vi "drawStrokeLines.vi"(0 "picture":picture, 1 "line endpoints":cluster{"x":i16, "y":i16}[](array[cluster]), 2 "fill?(F)":bool, 3 "color(black)":u32(colorbox), 4 "stroke":T1, 5 "error in (no error)":errorcluster, 9 "strokeLength":i32=5, 11 "black in B/W?(T)":bool=TRUE) -> (14 "new picture":picture, 19 "error out":errorcluster)   [LabVIEW 2016, in "Graphics.lvclass"]
doc: "Draws multiple connected lines into a picture."
uses:
  <resource>/Framework/Providers/Open_GDS/UML/Graphics_class/Graphics.lvclass
  <resource>/Framework/Providers/Open_GDS/UML/Graphics_class/StrokeType.ctl
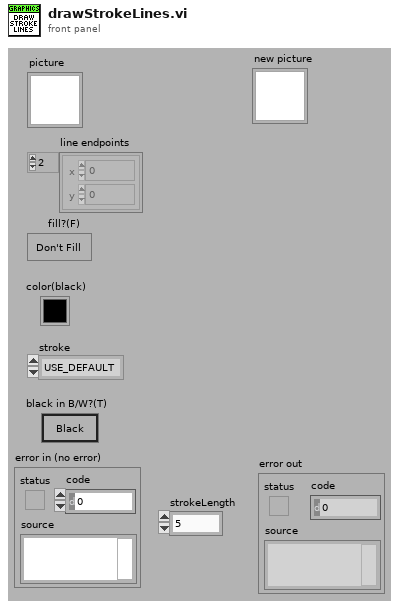
[diagram p1: front panel]
types:
  T1 = typedef "Graphics.lvclass/StrokeType.ctl" = enum16{"USE_DEFAULT", "SOLID", "DOTTED"}
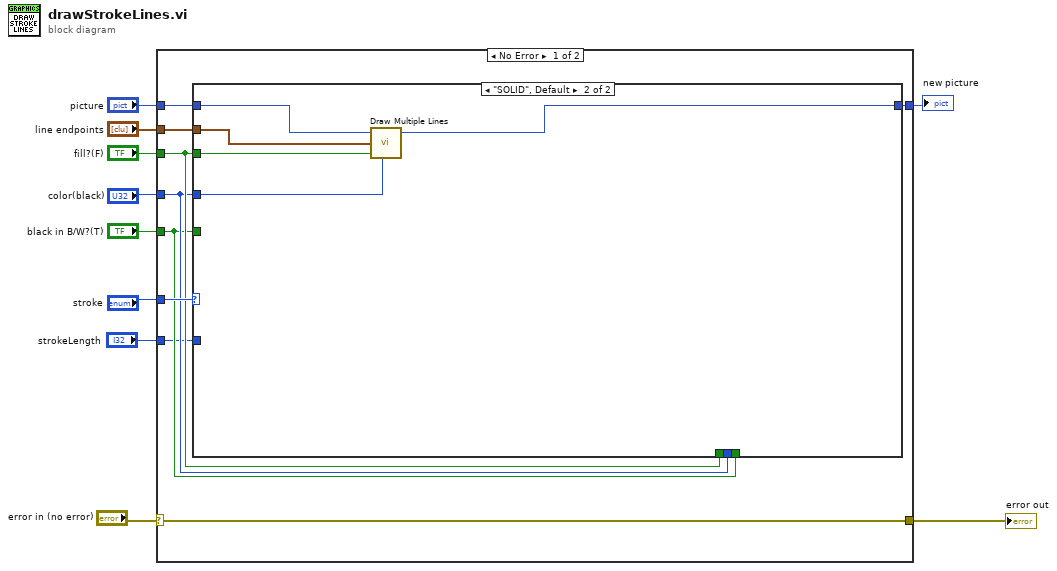
[diagram p0: block diagram]
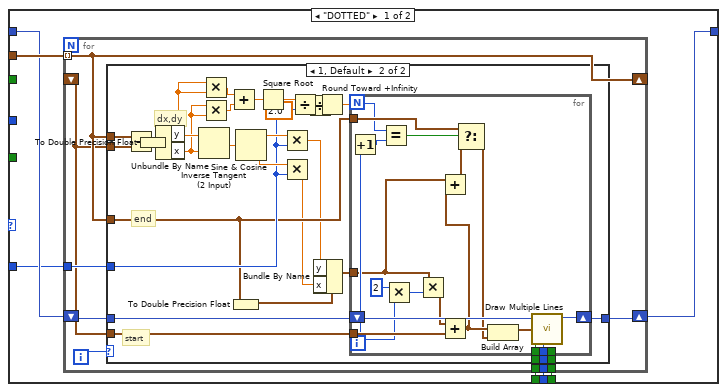
[diagram p2: hidden frame]
diagram:
  n1 = case shown="No Error" "error in (no error)" {
    selector: "error in (no error)" -> [w15 w90]
    tunnel: "picture" -> [w19 w89]
    tunnel: [w18 w89] -> w9
    tunnel: "fill?(F)" -> [w14 _]
    tunnel: "line endpoints" -> [w17 _]
    tunnel: "black in B/W?(T)" -> [w12 _]
    tunnel: "color(black)" -> [w13 _]
    tunnel: "stroke" -> [w16 _]
    tunnel: [w15 w90] -> w2
    tunnel: "strokeLength" -> [w11 _]
    frame No Error {
      n2 = case shown="\"SOLID\", Default" w16 {
        tunnel: w19 -> [w24 w88]
        tunnel: [w25 w87] -> w18
        tunnel: w14 -> [_ w86]
        tunnel: w17 -> [w26 w85]
        tunnel: w12 -> [_ _]
        tunnel: w13 -> [_ w84]
        tunnel: w14 -> [w23 _]
        tunnel: w13 -> [w22 _]
        tunnel: w12 -> [w21 _]
        tunnel: w11 -> [w20 _]
        frame "DOTTED" {
          n3 = for {
            shift-right: [w28] -> _
            shift-left: _ -> [w27]
            tunnel: w26 -> [w28] mode=indexing
            shift-right: [w34] -> w25
            shift-left: w24 -> [w33]
            tunnel: w23 -> [w32]
            tunnel: w22 -> [w31]
            tunnel: w21 -> [w30]
            tunnel: w20 -> [w29]
            i -> [w35]
            n4 = case shown="1, Default" w35 {
              tunnel: w28 -> [_ w44]
              tunnel: [w36 w57] -> w34
              tunnel: w33 -> [w36 w58]
              tunnel: w32 -> [_ w65]
              tunnel: w31 -> [_ w64]
              tunnel: w30 -> [_ w63]
              tunnel: w27 -> [_ w62]
              tunnel: w29 -> [_ w50]
              tunnel: w28 -> [_ w46]
              tunnel: w27 -> [_ w45]
              frame 0 {
              }
              frame 1, Default {
                # "start"
                # "end"
                # "dx,dy"
                n5 = Subtract(x=w46, y=w45) -> (x-y=w47:cluster{"x":i16, "y":i16})
                n6 = To Double Precision Float(number=w47) -> (double precision float=w38:cluster{"x":dbl, "y":dbl})
                n7 = Unbundle By Name(w38) -> ("y"=w56:dbl, "x"=w55:dbl)
                n8 = Inverse Tangent (2 Input)(1:w55, 2:w56) -> (0:w61:dbl)
                n9 = Multiply(x=w56, y=w56) -> (x*y=w53:dbl)
                n10 = Multiply(x=w55, y=w55) -> (x*y=w54:dbl)
                n11 = Add(x=w53, y=w54) -> (x+y=w52:dbl)
                n12 = To Double Precision Float(number=w44) -> (double precision float=w37:cluster{"x":dbl, "y":dbl})
                n13 = Sine & Cosine(0:w61) -> (1:w60:dbl, 2:w59:dbl)
                n14 = Square Root(x=w52) -> (sqrt(x)=w51:dbl)
                n15 = Multiply(x=w60, y=w50) -> (x*y=w42:dbl)
                n16 = Multiply(x=w59, y=w50) -> (x*y=w41:dbl)
                n17 = Divide(x=w51, y=w50) -> (x/y=w49:dbl)
                n18 = Divide(x=w49, y=2.0) -> (x/y=w40:dbl)
                n19 = Bundle By Name(cluster=w37, "y"=w42, "x"=w41) -> (w43:cluster{"x":dbl, "y":dbl})
                n20 = Round Toward +Infinity(x=w40) -> (ceil(x): smallest int >= x=w48:dbl)
                n21 = for {
                  N: w48 -> [w72]
                  tunnel: w65 -> [w83]
                  tunnel: w64 -> [w82]
                  tunnel: w63 -> [_]
                  tunnel: w62 -> [w79]
                  shift-right: [w77] -> w57
                  shift-left: w58 -> [w78]
                  tunnel: w43 -> [w67]
                  tunnel: w44 -> [w81]
                  i -> [w73]
                  n22 = Increment(x=w73) -> (x+1=w74:i32)
                  n23 = Equal?(x=w72, y=w74) -> (x = y?=w71:bool)
                  n24 = Multiply(x=2, y=w73) -> (x*y=w66:i32)
                  n25 = Multiply(x=w67, y=w66) -> (x*y=w68:cluster{"x":dbl, "y":dbl})
                  n26 = Add(x=w68, y=w79) -> (x+y=w76:cluster{"x":dbl, "y":dbl})
                  n27 = Add(x=w67, y=w76) -> (x+y=w69:cluster{"x":dbl, "y":dbl})
                  n28 = Select(t=w81, s=w71, f=w69) -> (s? t:f=w70:cluster{"x":dbl, "y":dbl})
                  n29 = Build Array(w76, w70) -> (w80:cluster{"x":dbl, "y":dbl}[])
                  n30 = call <vilib>:"Draw Multiple Lines.vi"("picture"=w78, "line endpoints"=w80, "fill?(F)"=w83, "color(black)"=w82) -> ("new picture"=w77:picture)  [unwired: 1 in, 4 out]
                }
              }
            }
          }
        }
        frame "SOLID", Default {
          n31 = call <vilib>:"Draw Multiple Lines.vi"("picture"=w88, "line endpoints"=w85, "fill?(F)"=w86, "color(black)"=w84) -> ("new picture"=w87:picture)  [unwired: 1 in, 4 out]
        }
      }
    }
    frame Error {
    }
  }
  "new picture" <- w9
  "error out" <- w2
